vi "ke37xx Line Synchronization.vi"(0 "VISA Resource Name":refnum<visa-resource-name>, 7 "Line Sync Enabled (F: Disabled)":bool, 11 "error in (no error)":errorcluster) -> (4 "VISA Resource Name Out":refnum<visa-resource-name>, 15 "error out":errorcluster)   [LabVIEW 2009, in "Keithley 3700 Series.lvlib"]
doc: "This VI controls whether line sync is used during measurements. When enabled, the system will synchronize a trigger to the main power line crossings. This VI only applies when the measurement function is DC Volts, DC Current, 2-Wire Ohms, 4-Wire Ohms, Temperature, or Continuity. All other measurement functions will generate an error if this VI is run."
uses:
  <instrlib>/Keithley 3706/Keithley 3700 Series.lvlib
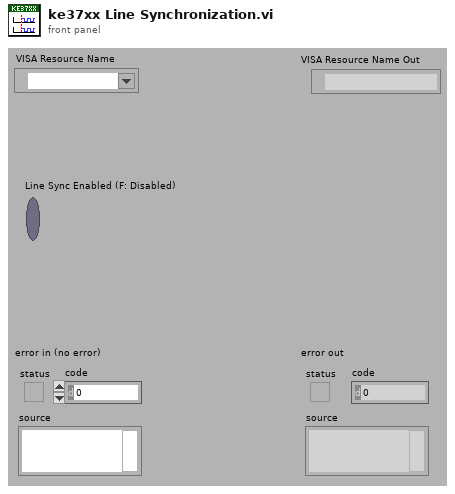
[diagram p1: front panel]
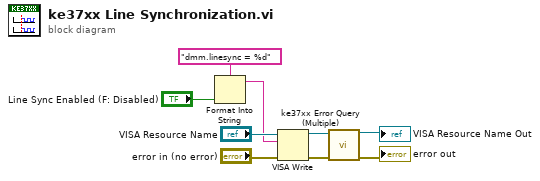
[diagram p0: block diagram]
diagram:
  n1 = Format Into String(format string="dmm.linesync = %d" ("write buffer"), "Line Sync Enabled (F: Disabled)") -> (resulting string=w2:string)  [unwired: 2 in, 1 out]
  n2 = VISA Write(VISA resource name="VISA Resource Name", write buffer=w2, error in (no error)="error in (no error)") -> (VISA resource name out=w5:refnum<visa-resource-name>, error out=w4:errorcluster)  [unwired: 1 out]
  n3 = call <instrlib>:"ke37xx Error Query (Multiple).vi"("VISA resource name"=w5, "error in (no error)"=w4) -> ("VISA resource name out"=→"VISA Resource Name Out":refnum<visa-resource-name>, "error out"=→"error out":errorcluster)  [unwired: 12 out]
